vi "IDC.vi"(5 "Axis(X,Y)":string, 6 "Program Number":string, 7 "baud rate (9600)":u32=115200 caption="보 전송속도(9600)", 8 "Port":refnum<visa-resource-name>="COM4" caption="VISA 리소스 이름") -> (0 "Error Out":errorcluster caption="에러 출력", 3 "VISA out":refnum<visa-resource-name>, 4 "IDC Information":string)   [LabVIEW 2010]
uses:
  <vilib>/Instr/_visa.llb/VISA Flush IO Buffer Mask.ctl
  <vilib>/Instr/_visa.llb/VISA Configure Serial Port (Instr).vi
panel:
  out "Commend Count":u32
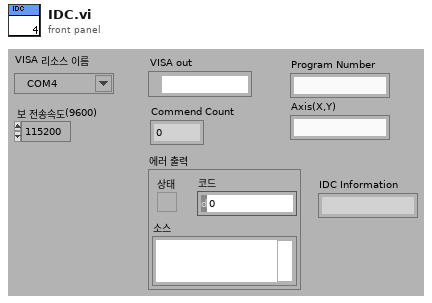
[diagram p1: front panel]
types:
  T1 = typedef "VISA Flush IO Buffer Mask.ctl" = u16
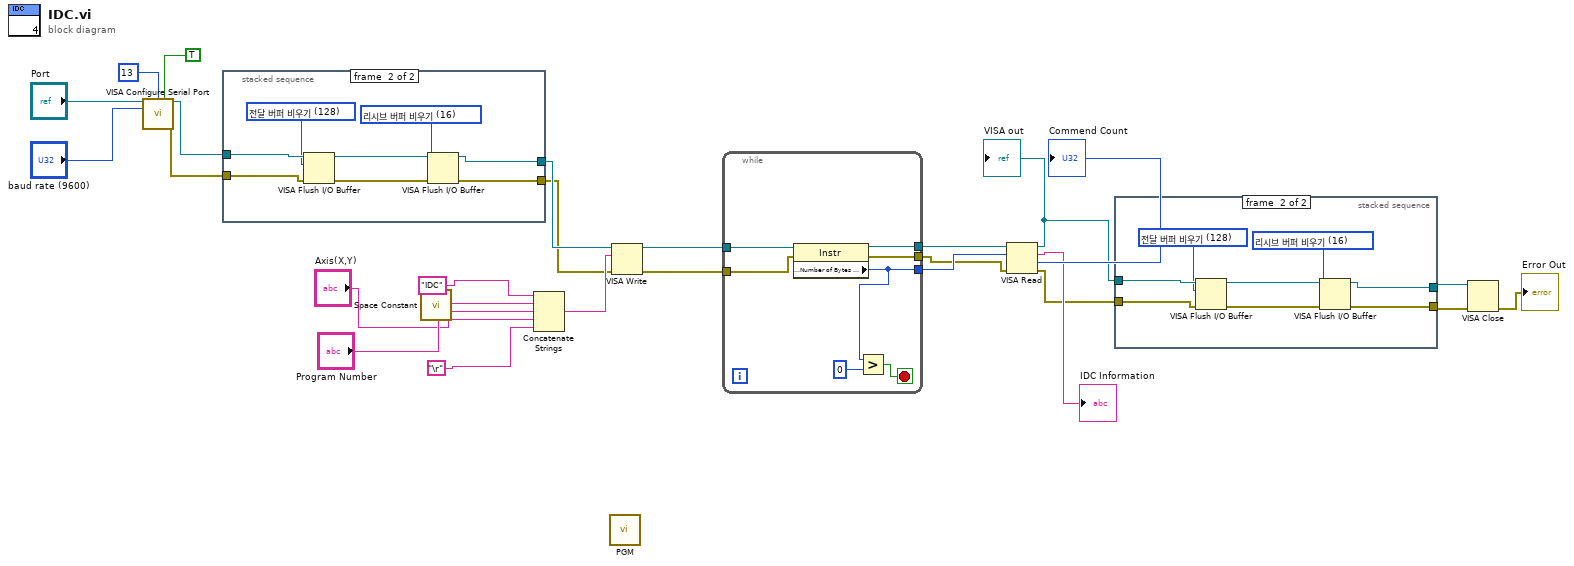
[diagram p0: block diagram]
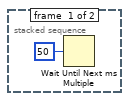
[diagram p2: hidden frame]
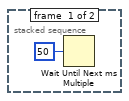
[diagram p3: hidden frame]
diagram:
  n1 = call-poly "VISA Configure Serial Port"("VISA resource name"="Port", "termination char\n(0xA = '\\n' = LF)"=i16 13 ("termination char\n(0xA = '\\n' = LF)"), "Enable Termination\nChar (T)"=TRUE ("Enable Termination\nChar (T)"), "baud rate (9600)"="baud rate (9600)") -> ("VISA resource name out"=w9:refnum<visa-resource-name>, "error out"=w8:errorcluster)  [unwired: 10 in]
  n2 = stacked-sequence {
    tunnel: w9 -> [_ w35]
    tunnel: w8 -> [_ w34]
    tunnel: [_ w30] -> w7
    tunnel: [_ w29] -> w6
    frame #0 {
      n3 = Wait Until Next ms Multiple(millisecond multiple=u32 50 ("ms 배수")) -> ()  [unwired: 1 out]
    }
    frame #1 {
      w28 = T1 16 items=["리시브 버퍼 비우기"=16, "전달 버퍼 디바이스에 쓰기"=32, "리시브 버퍼 비우기(I/O 없음)"=64, "전달 버퍼 비우기"=128] ("Mask")
      w33 = T1 128 items=["리시브 버퍼 비우기"=16, "전달 버퍼 디바이스에 쓰기"=32, "리시브 버퍼 비우기(I/O 없음)"=64, "전달 버퍼 비우기"=128] ("Mask")
      n4 = VISA Flush I/O Buffer(VISA resource name=w35, mask (16)=w33, error in (no error)=w34) -> (VISA resource name out=w32:refnum<visa-resource-name>, error out=w31:errorcluster)
      n5 = VISA Flush I/O Buffer(VISA resource name=w32, mask (16)=w28, error in (no error)=w31) -> (VISA resource name out=w30:refnum<visa-resource-name>, error out=w29:errorcluster)
    }
  }
  n6 = call <vilib>:"Space Constant.vi"() -> ("String"=w24:string)
  n7 = Concatenate Strings("IDC", w24, "Axis(X,Y)", "Program Number", "\r") -> (w25:string)
  n8 = call <userlib>:"PGM.vi"() -> ()  [unwired: 3 in, 2 out]
  n9 = VISA Write(VISA resource name=w7, write buffer=w25, error in (no error)=w6) -> (VISA resource name out=w23:refnum<visa-resource-name>, error out=w22:errorcluster)  [unwired: 1 out]
  n10 = while {
    tunnel: w23 -> [w42]
    tunnel: w22 -> [w41]
    tunnel: [w40] -> w21
    tunnel: [w37] -> w20
    tunnel: [w39] -> w19
    stop <- w38 stop-if-true
    n11 = property class="Instr"(reference=w42, error in=w41) -> (reference out=w40:refnum<visa-resource-name>, error out=w39:errorcluster, "Serial Settings:Number of Bytes at Serial Port"=w37:u32)
    n12 = Greater?(x=w37, y=u32 0) -> (0:w38:bool)
  }
  n13 = VISA Read(VISA resource name=w21, byte count=w20, error in (no error)=w19) -> (VISA resource name out=w5:refnum<visa-resource-name>, read buffer=→"IDC Information":string, return count=→"Commend Count":u32, error out=w4:errorcluster)
  "VISA out" <- w5
  n14 = stacked-sequence {
    tunnel: w5 -> [_ w51]
    tunnel: w4 -> [_ w50]
    tunnel: [_ w46] -> w3
    tunnel: [_ w45] -> w2
    frame #0 {
      n15 = Wait Until Next ms Multiple(millisecond multiple=u32 50 ("ms 배수")) -> ()  [unwired: 1 out]
    }
    frame #1 {
      w44 = T1 16 items=["리시브 버퍼 비우기"=16, "전달 버퍼 디바이스에 쓰기"=32, "리시브 버퍼 비우기(I/O 없음)"=64, "전달 버퍼 비우기"=128] ("Mask")
      w49 = T1 128 items=["리시브 버퍼 비우기"=16, "전달 버퍼 디바이스에 쓰기"=32, "리시브 버퍼 비우기(I/O 없음)"=64, "전달 버퍼 비우기"=128] ("Mask")
      n16 = VISA Flush I/O Buffer(VISA resource name=w51, mask (16)=w49, error in (no error)=w50) -> (VISA resource name out=w48:refnum<visa-resource-name>, error out=w47:errorcluster)
      n17 = VISA Flush I/O Buffer(VISA resource name=w48, mask (16)=w44, error in (no error)=w47) -> (VISA resource name out=w46:refnum<visa-resource-name>, error out=w45:errorcluster)
    }
  }
  n18 = VISA Close(VISA resource name=w3, error in (no error)=w2) -> (error out=→"Error Out":errorcluster)
